vi "AppKeyPath.vi"(8 "error in (no error)":errorcluster, 11 "FileName":string) -> (0 "error out":errorcluster, 2 "exists?":bool, 3 "AppKeyPath":path)   [LabVIEW 2019]
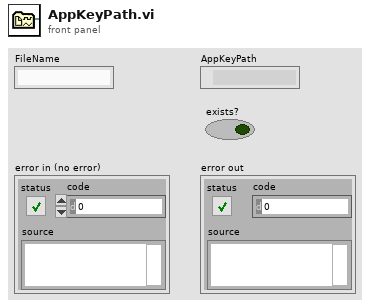
[diagram p1: front panel]
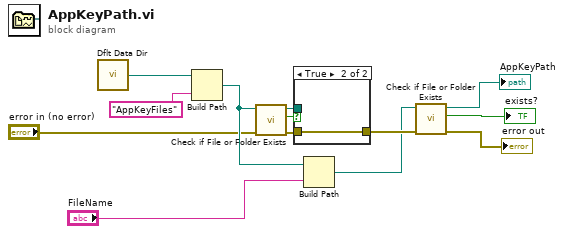
[diagram p0: block diagram]
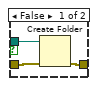
[diagram p2: hidden frame]
diagram:
  n1 = call <vilib>:"Dflt Data Dir.vi"() -> ("App:Default Data Directory"=w9:path)
  n2 = Build Path(base path=w9, name or relative path="AppKeyFiles") -> (appended path=w13:path)
  n3 = call <vilib>:"Check if File or Folder Exists.vi"("error in (no error)"="error in (no error)", "path"=w13) -> ("error out"=w12:errorcluster, "file or folder exists?"=w10:bool, "dup path"=w11:path)  [unwired: 7 in]
  n4 = case shown="True" w10 {
    tunnel: w11 -> [w16 _]
    tunnel: w12 -> [w15 w17]
    tunnel: [w14 w17] -> w7
    frame False {
      n5 = Create Folder(path (use dialog)=w16, error in=w15) -> (error out=w14:errorcluster)  [unwired: 1 in, 2 out]
    }
    frame True {
    }
  }
  n6 = Build Path(base path=w13, name or relative path="FileName") -> (appended path=w2:path)
  n7 = call <vilib>:"Check if File or Folder Exists.vi"("error in (no error)"=w7, "path"=w2) -> ("error out"=→"error out":errorcluster, "file or folder exists?"=→"exists?":bool, "dup path"=→"AppKeyPath":path)  [unwired: 7 in]
